vi "Read String.vi"(8 "error in (no error)":errorcluster, 11 "Modbus in":refnum<class "Modbus.lvclass">) -> (0 "error out":errorcluster, 1 "Bytes Read":i32, 2 "String Read":string, 3 "Modbus out":refnum<class "Modbus.lvclass">)   [LabVIEW 2018, in "Modbus.lvclass"]
doc: "Modbus.lvclass:Read String.vi\n\nThis reads a set of channels over Modbus and flattens the resulting double-precision numbers to a string.\n\nInstrument Communication Module Version 1.0\nJanuary, 2018 Original Code Consulting David Thomson\n www.originalcode.com"
uses:
  Modbus.lvclass
  Modbus.lvclass/Modbus.ctl
  Modbus Master.lvclass
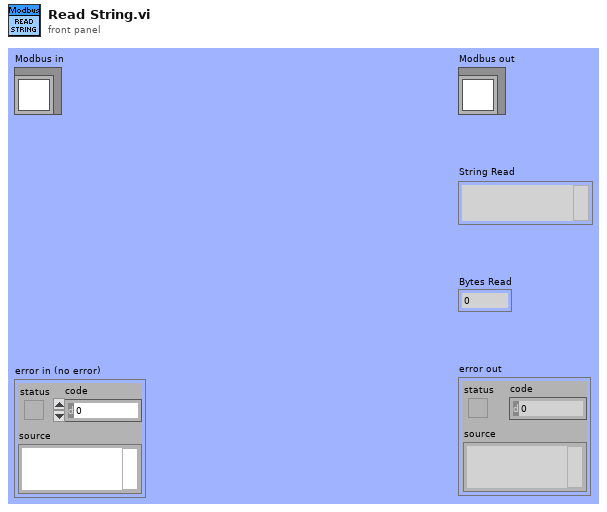
[diagram p1: front panel]
types:
  T1 = typedef "ICM Modbus Data Type.ctl" = enum16{"Boolean", "U16 (unsigned 16bit Int)", "I16 (signed 16bit Int)", "U32 (unsigned 32bit Int)", "I32 (signed 32bit Int)", "Real (Single 32bit)"}
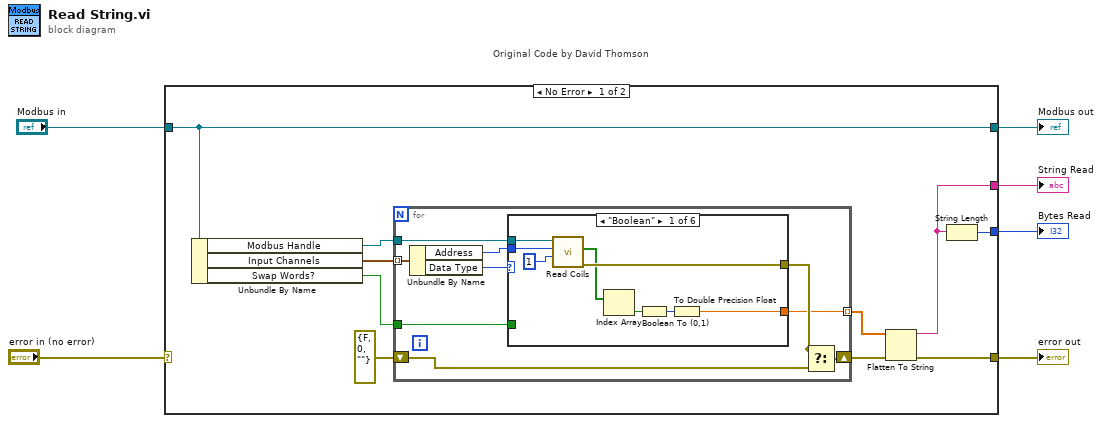
[diagram p0: block diagram]
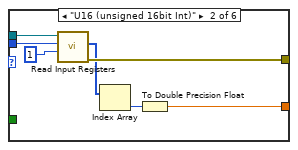
[diagram p2: hidden frame]
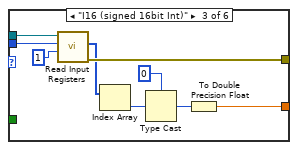
[diagram p3: hidden frame]
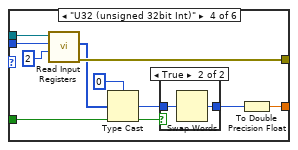
[diagram p4: hidden frame]
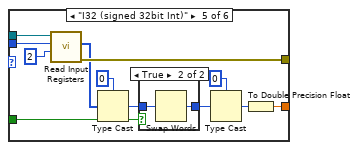
[diagram p6: hidden frame]
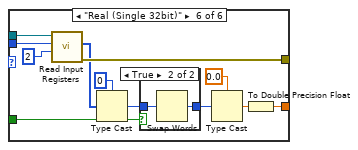
[diagram p8: hidden frame]
diagram:
  n1 = case "Original Code by David Thomson" shown="No Error" "error in (no error)" {
    selector: "error in (no error)" -> [_ w93]
    tunnel: [w12 w94] -> w5
    tunnel: "Modbus in" -> [w12 w94]
    tunnel: [w9 w93] -> w3
    tunnel: [w8 _] -> w2
    tunnel: [w7 _] -> w1
    frame No Error {
      n2 = Unbundle By Name(w12) -> ("Modbus Handle"=w14:refnum<class "Modbus Master.lvclass">, "Input Channels"=w15:cluster{"Data Type":T1, "Address":u16}[], "Swap Words?"=w13:bool)
      n3 = for {
        tunnel: w15 -> [w25] mode=indexing
        shift-right: [w24] -> w10
        shift-left: errorcluster {"status"=FALSE, "code"=0, "source"=""} ("error out") -> [w23]
        tunnel: w14 -> [w21]
        tunnel: w13 -> [w18]
        tunnel: [w17] -> w11 mode=indexing
        n4 = Unbundle By Name(w25) -> ("Address"=w20:u16, "Data Type"=w19:T1)
        n5 = case shown="\"Boolean\"" w19 {
          tunnel: w21 -> [w33 w40 w49 w59 w74 w89]
          tunnel: w20 -> [w32 w39 w48 w58 w73 w88]
          tunnel: [w31 w38 w47 w57 w72 w87] -> w22
          tunnel: [w27 w35 w45 w56 w71 w86] -> w17
          tunnel: w18 -> [_ _ _ w50 w63 w78]
          frame "Boolean" {
            n6 = call-dynamic "Read Coils.vi"("number of coils"=u16 1 ("number of inputs"), "starting address"=w32, "Modbus master in"=w33) -> ("error out"=w31:errorcluster, "coil values"=w30:bool[])  [unwired: 6 in, 1 out]
            n7 = Index Array(array=w30) -> (element=w29:bool)  [unwired: 1 in]
            n8 = Boolean To (0,1)(Boolean=w29) -> (0, 1=w28:i16)
            n9 = To Double Precision Float(number=w28) -> (double precision float=w27:dbl)
          }
          frame "U16 (unsigned 16bit Int)" {
            n10 = call-dynamic "Read Input Registers.vi"("number of input registers"=u16 1 ("number of inputs"), "starting address"=w39, "Modbus master in"=w40) -> ("error out"=w38:errorcluster, "register values"=w37:u16[])  [unwired: 6 in, 1 out]
            n11 = Index Array(array=w37) -> (element=w36:u16)  [unwired: 1 in]
            n12 = To Double Precision Float(number=w36) -> (double precision float=w35:dbl)
          }
          frame "I16 (signed 16bit Int)" {
            n13 = call-dynamic "Read Input Registers.vi"("number of input registers"=u16 1 ("number of inputs"), "starting address"=w48, "Modbus master in"=w49) -> ("error out"=w47:errorcluster, "register values"=w46:u16[])  [unwired: 6 in, 1 out]
            n14 = Index Array(array=w46) -> (element=w44:u16)  [unwired: 1 in]
            n15 = Type Cast(type=i16 0, x=w44) -> (*(type *) &x=w42:i16)
            n16 = To Double Precision Float(number=w42) -> (double precision float=w45:dbl)
          }
          frame "U32 (unsigned 32bit Int)" {
            n17 = call-dynamic "Read Input Registers.vi"("number of input registers"=u16 2 ("number of inputs"), "starting address"=w58, "Modbus master in"=w59) -> ("error out"=w57:errorcluster, "register values"=w53:u16[])  [unwired: 6 in, 1 out]
            n18 = Type Cast(type=u32 0, x=w53) -> (*(type *) &x=w52:u32)
            n19 = case shown="True" w50 {
              tunnel: w52 -> [w60 w62]
              tunnel: [w60 w61] -> w51
              frame False {
              }
              frame True {
                n20 = Swap Words(1:w62) -> (0:w61:u32)
              }
            }
            n21 = To Double Precision Float(number=w51) -> (double precision float=w56:dbl)
          }
          frame "I32 (signed 32bit Int)" {
            n22 = call-dynamic "Read Input Registers.vi"("number of input registers"=u16 2 ("number of inputs"), "starting address"=w73, "Modbus master in"=w74) -> ("error out"=w72:errorcluster, "register values"=w68:u16[])  [unwired: 6 in, 1 out]
            n23 = Type Cast(type=u32 0, x=w68) -> (*(type *) &x=w64:u32)
            n24 = case shown="True" w63 {
              tunnel: w64 -> [w75 w77]
              tunnel: [w75 w76] -> w65
              frame False {
              }
              frame True {
                n25 = Swap Words(1:w77) -> (0:w76:u32)
              }
            }
            n26 = Type Cast(type=0, x=w65) -> (*(type *) &x=w67:i32)
            n27 = To Double Precision Float(number=w67) -> (double precision float=w71:dbl)
          }
          frame "Real (Single 32bit)" {
            n28 = call-dynamic "Read Input Registers.vi"("number of input registers"=u16 2 ("number of inputs"), "starting address"=w88, "Modbus master in"=w89) -> ("error out"=w87:errorcluster, "register values"=w83:u16[])  [unwired: 6 in, 1 out]
            n29 = Type Cast(type=u32 0, x=w83) -> (*(type *) &x=w79:u32)
            n30 = case shown="True" w78 {
              tunnel: w79 -> [w90 w92]
              tunnel: [w90 w91] -> w80
              frame False {
              }
              frame True {
                n31 = Swap Words(1:w92) -> (0:w91:u32)
              }
            }
            n32 = Type Cast(type=sgl 0.0, x=w80) -> (*(type *) &x=w82:sgl)
            n33 = To Double Precision Float(number=w82) -> (double precision float=w86:dbl)
          }
        }
        n34 = Select(t=w22, s=w22, f=w23) -> (s? t:f=w24:errorcluster)
      }
      n35 = Flatten To String(anything=w11, error in (no error)=w10) -> (data string=w7:string, error out=w9:errorcluster)  [unwired: 2 in, 1 out]
      n36 = String Length(string=w7) -> (length=w8:i32)
    }
    frame Error {
    }
  }
  "error out" <- w3
  "Modbus out" <- w5
  "Bytes Read" <- w2
  "String Read" <- w1
